vi "S2.vi"(1 "Input array":bool[](array[boolean])) -> (0 "Array":bool[](array[boolean]))   [LabVIEW 2013]
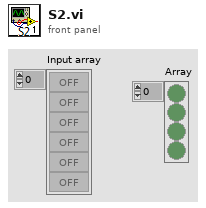
[diagram p1: front panel]
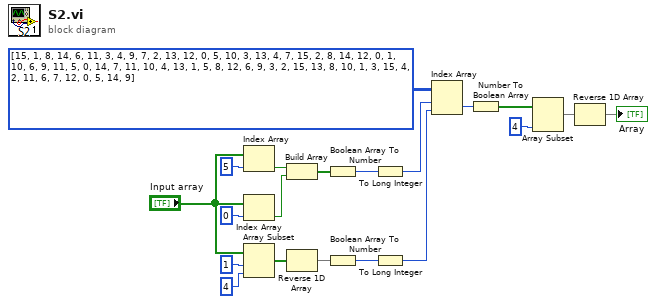
[diagram p0: block diagram]
diagram:
  n1 = Index Array(array="Input array", index=5) -> (element=w5:bool)
  n2 = Index Array(array="Input array", index=0) -> (element=w4:bool)
  n3 = Array Subset(array="Input array", index=1, length=4) -> (w2:bool[])
  n4 = Build Array(w5, w4) -> (w3:bool[])
  n5 = Reverse 1D Array(array=w2) -> (reversed array=w1:bool[])
  n6 = Boolean Array To Number(Boolean array=w3) -> (number=w12:u32)
  n7 = Boolean Array To Number(Boolean array=w1) -> (number=w11:u32)
  n8 = To Long Integer(number=w12) -> (32bit integer=w8:i32)
  n9 = To Long Integer(number=w11) -> (32bit integer=w7:i32)
  n10 = Index Array(array=u8[][] [[15, 1, 8, 14, 6, 11, 3, 4, 9, 7, 2, 13, 12, 0, 5, 10], [3, 13, 4, 7, 15, 2, 8, 14, 12, 0, 1, 10, 6, 9, 11, 5], [0, 14, 7, 11, 10, 4, 13, 1, 5, 8, 12, 6, 9, 3, 2, 15], [13, 8, 10, 1, 3, 15, 4, 2, 11, 6, 7, 12, 0, 5, 14, 9]], index (row)=w8, index (col)=w7) -> (element=w17:u8)
  n11 = Number To Boolean Array(number=w17) -> (Boolean array=w16:bool[])
  n12 = Array Subset(array=w16, length=4) -> (w6:bool[])  [unwired: 1 in]
  n13 = Reverse 1D Array(array=w6) -> (reversed array=→"Array":bool[])
